vi "Initialize.vi"(8 "error in":errorcluster, 11 "NOAA Wide in":refnum<class "NOAA Wide.lvclass">) -> (0 "error out":errorcluster, 3 "NOAA Wide out":refnum<class "NOAA Wide.lvclass">)   [LabVIEW 2015, in "NOAA Wide.lvclass"]
uses:
  NOAA Wide.lvclass
  DMA.lvclass/DMA.ctl
  Accessors/Write ri.vi
  Accessors/Write ro.vi
  Accessors/Write Leff.vi
  DMA.lvclass
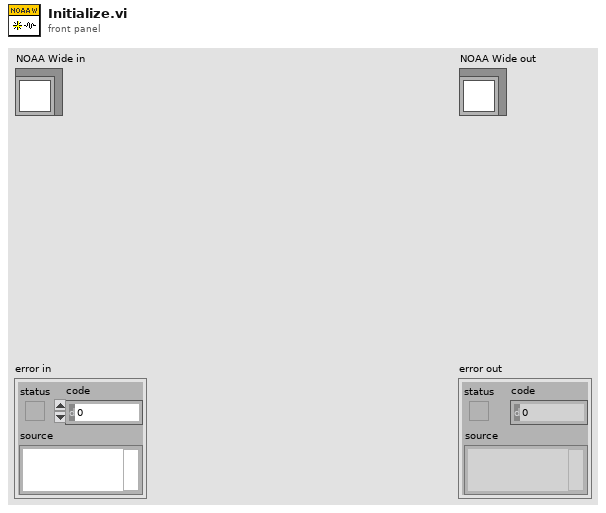
[diagram p1: front panel]
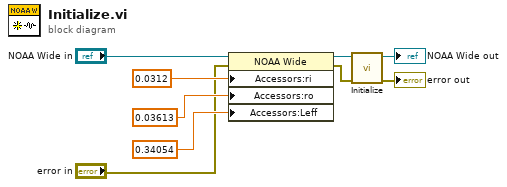
[diagram p0: block diagram]
diagram:
  n1 = property class="NOAA Wide"(reference="NOAA Wide in", error in="error in", "Accessors:ri"=0.0312 ("ri"), "Accessors:ro"=0.03613 ("ro"), "Accessors:Leff"=0.34054 ("Leff")) -> (reference out=w6:refnum<class "NOAA Wide.lvclass">, error out=w1:errorcluster)
  n2 = call-parent "Initialize.vi"("error in"=w1, "DMA in"=w6) -> ("error out"=→"error out":errorcluster, "DMA out"=→"NOAA Wide out":refnum<class "NOAA Wide.lvclass">)  [unwired: 8 in]
